vi "DS345_BurstMode.ProcEvents.vi"(0 "i ref in":refnum<vi>, 5 "error in (no error)":errorcluster) -> (14 "i ref out":refnum<vi>, 19 "error out":errorcluster)   [LabVIEW 2014, in "DS345_BurstMode.lvlib"]
doc: "This method is used during the 1st frame of the process object to define the events the object will listen to. Add your own events here."
uses:
  DS345_BurstMode.lvlib
  CSCore/BaseProcess/BaseProcess.event definition.ctl
  CSCore/CAEObj/CAEObj.event definition.ctl
  CSCore/BaseProcess/BaseProcess.descriptor string definition.ctl
  CSCore/BaseProcess/BaseProcess.lvlib
  CSCore/CAEObj/CAEObj.lvlib
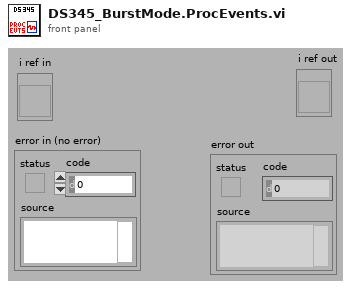
[diagram p1: front panel]
types:
  T1 = typedef "BaseProcess.lvlib/BaseProcess.event definition.ctl" = cluster{"CAEEvtDef":T2, "Data Descriptor":T3}
  T2 = typedef "CAEObj.lvlib/CAEObj.event definition.ctl" = cluster{"URL":string, "enable":bool, "ignoreResID":bool}
  T3 = typedef "BaseProcess.lvlib/BaseProcess.descriptor string definition.ctl" = string
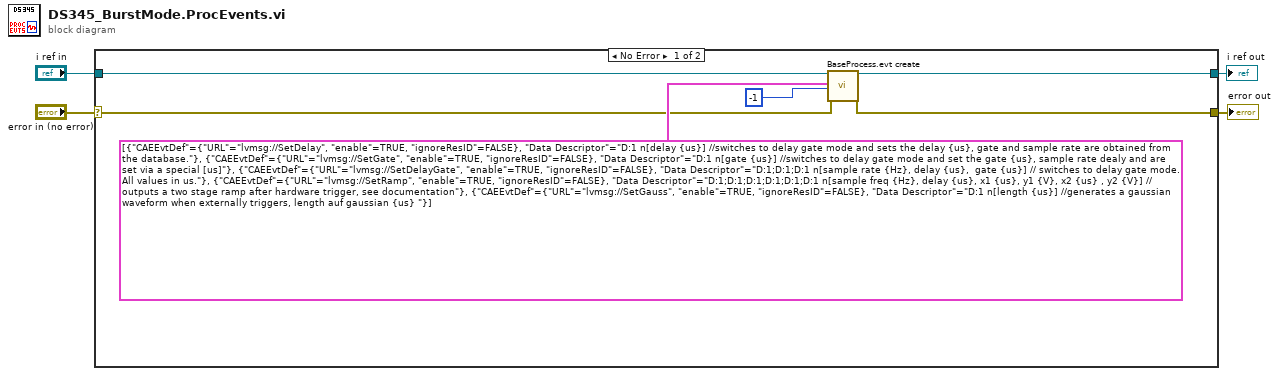
[diagram p0: block diagram]
diagram:
  n1 = case shown="No Error" "error in (no error)" {
    selector: "error in (no error)" -> [w5 w11]
    tunnel: "i ref in" -> [w10 w12]
    tunnel: [w9 w12] -> w3
    tunnel: [w8 w11] -> w2
    frame No Error {
      n2 = call "BaseProcess.evt create.vi"("i ref in"=w10, "newEvents"=T1[] [{"CAEEvtDef"={"URL"="lvmsg://SetDelay", "enable"=TRUE, "ignoreResID"=FALSE}, "Data Descriptor"="D:1 n[delay {us}] //switches to delay gate mode and sets the delay {us}, gate and sample rate are obtained from the database."}, {"CAEEvtDef"={"URL"="lvmsg://SetGate", "enable"=TRUE, "ignoreResID"=FALSE}, "Data Descriptor"="D:1 n[gate {us}] //switches to delay gate mode and set the gate {us}, sample rate dealy and are set via a special [us]"}, {"CAEEvtDef"={"URL"="lvmsg://SetDelayGate", "enable"=TRUE, "ignoreResID"=FALSE}, "Data Descriptor"="D:1;D:1;D:1 n[sample rate {Hz}, delay {us},  gate {us}] // switches to delay gate mode. All values in us."}, {"CAEEvtDef"={"URL"="lvmsg://SetRamp", "enable"=TRUE, "ignoreResID"=FALSE}, "Data Descriptor"="D:1;D:1;D:1;D:1;D:1;D:1 n[sample freq {Hz}, delay {us}, x1 {us}, y1 {V}, x2 {us} , y2 {V}] //outputs a two stage ramp after hardware trigger, see documentation"}, {"CAEEvtDef"={"URL"="lvmsg://SetGauss", "enable"=TRUE, "ignoreResID"=FALSE}, "Data Descriptor"="D:1 n[length {us}] //generates a gaussian waveform when externally triggers, length auf gaussian {us} "}] ("new events"), "ms timeout (10000)"=-1, "error in (no error)"=w5) -> ("i ref out"=w9:refnum<vi>, "error out"=w8:errorcluster)  [unwired: 12 in, 2 out]
    }
    frame Error {
    }
  }
  "i ref out" <- w3
  "error out" <- w2
